vi "SaveFromMemory.vi"(8 "error in (no error)":errorcluster, 10 "Data_2_Save":T1(array[cluster]), 11 "DBAL in":refnum<class "DBAL.lvclass">) -> (0 "error out":errorcluster, 3 "DBAL out":refnum<class "DBAL.lvclass">)   [LabVIEW 2020, in "Sgraph_lib_V1.lvlib" / "DBAL.lvclass"]
doc: "Must override!"
uses:
  DBAL.lvclass
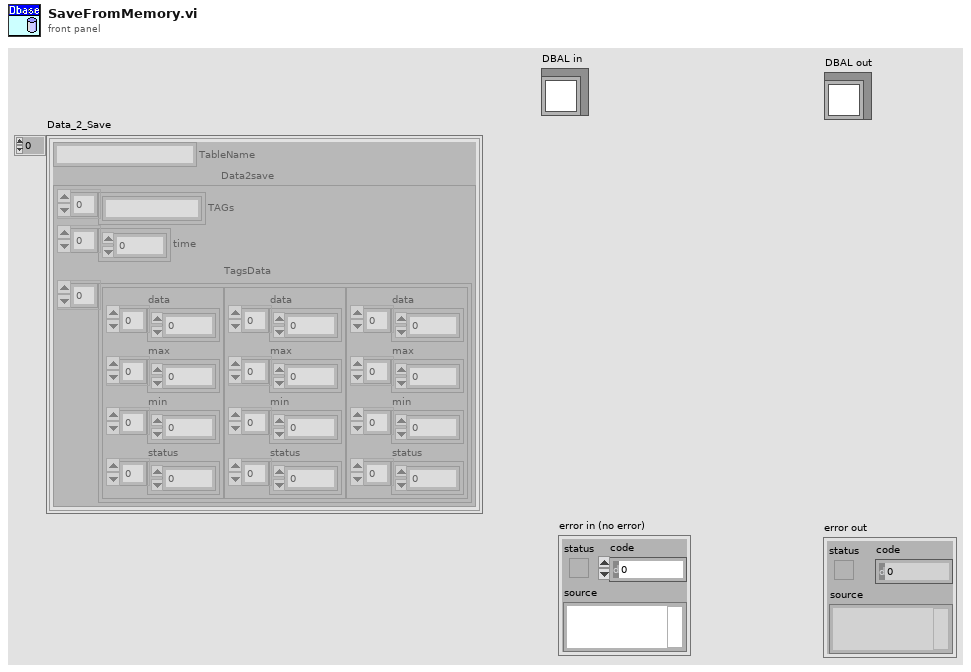
[diagram p1: front panel]
types:
  T1 = cluster{"TableName":string, "Data2save":cluster{"TAGs":string[], "time":dbl[], "TagsData":cluster{"data":dbl[], "max":dbl[], "min":dbl[], "status":u32[]}[]}}[]
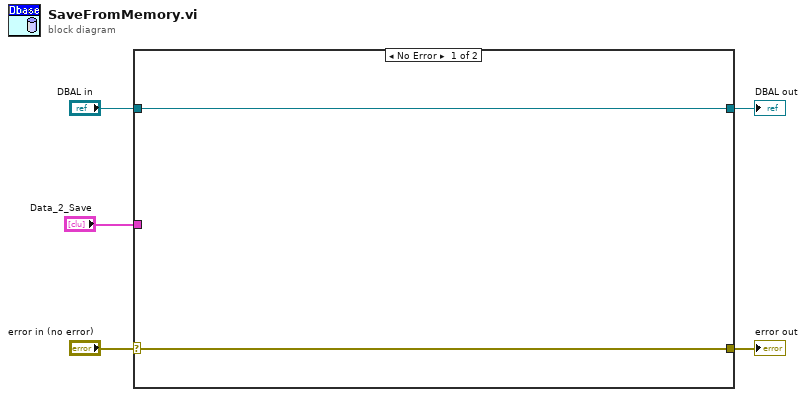
[diagram p0: block diagram]
diagram:
  n1 = case shown="No Error" "error in (no error)" {
    selector: "error in (no error)" -> [w6 w9]
    tunnel: [w6 w9] -> w4
    tunnel: [w7 w8] -> w2
    tunnel: "DBAL in" -> [w7 w8]
    tunnel: "Data_2_Save" -> [_ _]
    frame No Error {
    }
    frame Error {
    }
  }
  "error out" <- w4
  "DBAL out" <- w2
